vi "PowerMonitor Engine Driver.vi"(11 "Sequence Context":T2) -> (0 "error out":errorcluster)   [LabVIEW 2023, in "LTT_TeststandSteptypes.lvlib"]
uses:
  LTT_TeststandSteptypes.lvlib
  <vilib>/addons/TestStand/_TSLegacy.llb/LabVIEW Test - Sequence Context.ctl
  HardwareAbstractionLayer_LVOOP/Digital Input/DI_class/DI DAQ/Control/DI Step Control.ctl
  HardwareAbstractionLayer_LVOOP/PowerSupply/Control/PPS FGV Option.ctl
  Control/PowerData.ctl
  HardwareAbstractionLayer_LVOOP/Report/Report_class/Control/All Log Details.ctl
  HardwareAbstractionLayer_LVOOP/Report/Report_class/Control/UUT Test Info.ctl
  HardwareAbstractionLayer_LVOOP/Report/Report_class/Control/FE FRAME LOG.ctl
  HardwareAbstractionLayer_LVOOP/Report/Report_class/Control/FF FRAME LOG.ctl
  HardwareAbstractionLayer_LVOOP/Report/Report_class/Control/LIMIT TABLE.ctl
  HardwareAbstractionLayer_LVOOP/Report/Report_class/Control/ERROR LOG APPEND.ctl
  HardwareAbstractionLayer_LVOOP/Report/Report_class/Control/ERROR LOG.ctl
  HardwareAbstractionLayer_LVOOP/Report/Report_class/Control/FA FRAME LOG.ctl
  HardwareAbstractionLayer_LVOOP/Report/Report_class/Control/TEST RESULT LOG APPEND.ctl
  HardwareAbstractionLayer_LVOOP/Report/Report_class/Control/TEST RESULT LOG.ctl
  HardwareAbstractionLayer_LVOOP/Report/Report_class/Control/SYSTEM LOG.ctl
  HardwareAbstractionLayer_LVOOP/Report/Report_class/Control/Temperature LOG.ctl
  HardwareAbstractionLayer_LVOOP/Report/Report_class/Control/POWER STATUS.ctl
  HardwareAbstractionLayer_LVOOP/Report/Report_class/Control/CYCLE_DURATION_LOG.ctl
  Control/TimerStates.ctl
  GlobalVariable/GlobalVariableData.vi
  <vilib>/addons/TestStand/_TSUtility.llb/TestStand - Get Property Value (Number {Unsigned 32-bit Integer}).vi
  HardwareAbstractionLayer_LVOOP/Report/Report_class/Report.lvclass
  HardwareAbstractionLayer_LVOOP/Database/Database.lvclass
  HardwareAbstractionLayer_LVOOP/PowerSupply/PowerSupply.lvclass
  HardwareAbstractionLayer_LVOOP/Digital Input/DI_class/DI.lvclass
panel:
  in  "DI In":T1
  in  "stop":bool
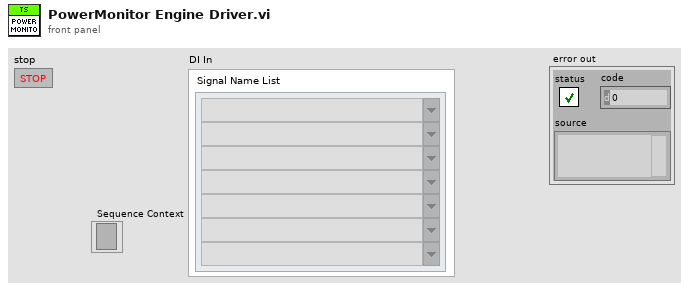
[diagram p1: front panel]
types:
  T1 = typedef "HardwareAbstractionLayer_LVOOP.lvlib/DI.lvclass/DI Step Control.ctl" = cluster{"Signal Name List":string[]}
  T2 = typedef "LabVIEW Test - Sequence Context.ctl" = refnum<k7>
  T3 = typedef "HardwareAbstractionLayer_LVOOP.lvlib/PowerSupply.lvclass/PPS FGV Option.ctl" = enum16{"Init Ref", "Get Ref", "Set Ref"}
  T4 = typedef "LTT_TeststandSteptypes.lvlib/PowerData.ctl" = cluster{"Chamber IP Ping":bool, "RAW_Power_Status":bool, "PDU1_Status_Instrument_Rack":bool, "PDU2_Status_PowerSupply_Rack_1":bool, "PDU3_Status_PowerSupply_Rack_2":bool}
  T5 = typedef "LTT_TeststandSteptypes.lvlib/TimerStates.ctl" = enum16{"Run", "Pause", "Reset"}
  T6 = typedef "HardwareAbstractionLayer_LVOOP.lvlib/Report.lvclass/All Log Details.ctl" = cluster{"UUT_TEST_INFO":T7, "FE_FRAME_LOG":T8, "FF_FRAME_LOG":T9, "LIMIT_TABLE":T10, "ERROR LOG Append":T11, "FA_FRAME_LOG":T13, "Socket No":u16, "TEST RESULT LOG Append":T14, "SYSTEM_LOG":T16, "Temperature log":T17, "POWER_STATUS":T18, "CYCLE_DURATION_LOG":T19}
  T7 = typedef "HardwareAbstractionLayer_LVOOP.lvlib/Report.lvclass/UUT Test Info.ctl" = cluster{"ID":string, "STATION_ID":string, "TEST_SOCKET_INDEX":string, "UUT_SERIAL_NUMBER":string, "TSW_VER":string, "VAL_SW_VER":string, "PROJECT_NAME":string, "PRODUCT_NAME":string, "PRODUCT_VARIANT":string, "TEST_NAME":string, "TEST_PHASE":string, "TEST_DESCRIPTION":string, "TEMP_CHAMBER_NAME":string, "START_DATE_TIME":string, "STOP_DATE_TIME ":string, "START_CYCLE_COUNT":string, "STOP_CYCLE_COUNT":string, "EXECUTION_TIME":string, "UUT_STATUS":string, "UUT_ERROR_CODE":string, "UUT_ERROR_MESSAGE":string, "TEST_SEQUENCE":string}
  T8 = typedef "HardwareAbstractionLayer_LVOOP.lvlib/Report.lvclass/FE FRAME LOG.ctl" = cluster{"ID":string, "UUT_TEST_INFO":string, "DATE_TIME":string, "CYCLE_NUMBER":string, "TEST_MODE":string, "CHAMBER_TEMP":string, "CAN_FRAME_RX":string, "Test Mode":u32, "LV_PPS_VOLTAGE":string, "LV_PPS_CURRENT":string, "HV_PPS_VOLTAGE":string, "HV_PPS_CURRENT":string, "SOCKET_NUMBER":string, "CAN_FRAME_RX_NO_OFF_BYTE":string}
  T9 = typedef "HardwareAbstractionLayer_LVOOP.lvlib/Report.lvclass/FF FRAME LOG.ctl" = cluster{"ID":string, "UUT_TEST_INFO":string, "DATE_TIME":string, "CYCLE_NUMBER":string, "TEST_MODE":string, "CAN_FRAME_RX":string, "CHAMBER_TEMP":string, "TestMode":u32, "SOCKET_NUMBER":string, "CAN_FRAME_RX_NO_OFF_BYTE":string}
  T10 = typedef "HardwareAbstractionLayer_LVOOP.lvlib/Report.lvclass/LIMIT TABLE.ctl" = cluster{"ID":string, "PRODUCT_NAME":string, "PRODUCT_VARIANT":string, "TEST_MODE":string, "PARAMETER_NAME":string, "COMPARISON_TYPE":string, "LOW_LIMIT":string, "HIGH_LIMIT":string, "UNIT":string, "ERROR_MESSSAGE":string, "SEVERITY":string}
  T11 = typedef "HardwareAbstractionLayer_LVOOP.lvlib/Report.lvclass/ERROR LOG APPEND.ctl" = T12[]
  T12 = typedef "HardwareAbstractionLayer_LVOOP.lvlib/Report.lvclass/ERROR LOG.ctl" = cluster{"ID":string, "UUT_TEST_INFO":string, "DATE_TIME":string, "CYCLE_NUMBER":string, "TEST_MODE":string, "SIGNAL_NAME":string, "SIGNAL_VALUE":string, "UNIT":string, "COMPARISON_VALUE":string, "ERROR_MESSAGE":string, "FRAME_TYPE":string, "LIMITID":string, "SOCKET_NUMBER":string}
  T13 = typedef "HardwareAbstractionLayer_LVOOP.lvlib/Report.lvclass/FA FRAME LOG.ctl" = cluster{"UUT_TEST_INFO":string, "CAN_FRAME_RX":string, "CAN_FRAME_RX_NO_OFF_BYTE":string}
  T14 = typedef "HardwareAbstractionLayer_LVOOP.lvlib/Report.lvclass/TEST RESULT LOG APPEND.ctl" = T15[]
  T15 = typedef "HardwareAbstractionLayer_LVOOP.lvlib/Report.lvclass/TEST RESULT LOG.ctl" = cluster{"ID":string, "UUT_TEST_INFO":string, "DATE_TIME":string, "CYCLE_NUMBER":string, "TEST_MODE":string, "SIGNAL_NAME":string, "SIGNAL_VALUE":string, "COMPARISON_VALUE":string, "ERROR_MESSAGE":string, "FRAME_TYPE":string, "LIMITID":string, "TEST_RESULT":string, "SOCKET_NUMBER":string}
  T16 = typedef "HardwareAbstractionLayer_LVOOP.lvlib/Report.lvclass/SYSTEM LOG.ctl" = cluster{"ID ":string, "DATE_TIME":string, "CYCLE_NUMBER":string, "TEST_MODE":string, "ERROR_MESSAGE":string}
  T17 = typedef "HardwareAbstractionLayer_LVOOP.lvlib/Report.lvclass/Temperature LOG.ctl" = cluster{"TEST_MODE":string, "CYCLE_NUMBER":string, "TEMPERATURE":cluster{"LV_PPS_TEMPERATURE":dbl, "HV_PPS1_TEMPERATURE":dbl, "HV_PPS2_TEMPERATURE":dbl, "HV_PPS3_TEMPERATURE":dbl, "HV_PPS4_TEMPERATURE":dbl, "HV_PPS5_TEMPERATURE":dbl, "HV_PPS6_TEMPERATURE":dbl, "CHAMBER_TEMPERATURE":dbl, "LOAD_U1_TEMPERATURE":dbl, "LOAD_V1_TEMPERATURE":dbl, "LOAD_W1_TEMPERATURE":dbl, "LOAD_U2_TEMPERATURE":dbl, "LOAD_V2_TEMPERATURE":dbl, "LOAD_W2_TEMPERATURE":dbl, "LOAD_U3_TEMPERATURE":dbl, "LOAD_V3_TEMPERATURE":dbl, "LOAD_W3_TEMPERATURE":dbl}, "Temperature Inrange":cluster{"LVPPS_Trip?":bool, "HVPPS1_Trip?":bool, "HVPPS2_Trip?":bool, "HVPPS3_Trip?":bool, "HVPPS4_Trip?":bool, "HVPPS5_Trip?":bool, "HVPPS6_Trip?":bool, "Chamber_Trip?":bool}}
  T18 = typedef "HardwareAbstractionLayer_LVOOP.lvlib/Report.lvclass/POWER STATUS.ctl" = cluster{"TEST_MODE":string, "CYCLE_NUMBER":string, "TYPE_POWER":string, "STATE":string}
  T19 = typedef "HardwareAbstractionLayer_LVOOP.lvlib/Report.lvclass/CYCLE_DURATION_LOG.ctl" = cluster{"CYCLE_NUMBER":string}
  T20 = typedef "HardwareAbstractionLayer_LVOOP.lvlib/Report.lvclass/Result FGV Data.ctl" = cluster{"Project Name":string, "Product Name":string, "Product Varient":string, "Test Name":string, "Test Phase":string, "Test Description":string, "Temp Chamber Name":string, "Schema":string, "Total No of Cycles":u32, "Current Cycle Number":u32, "Cycle Duration":u32, "Current Test Mode":string}
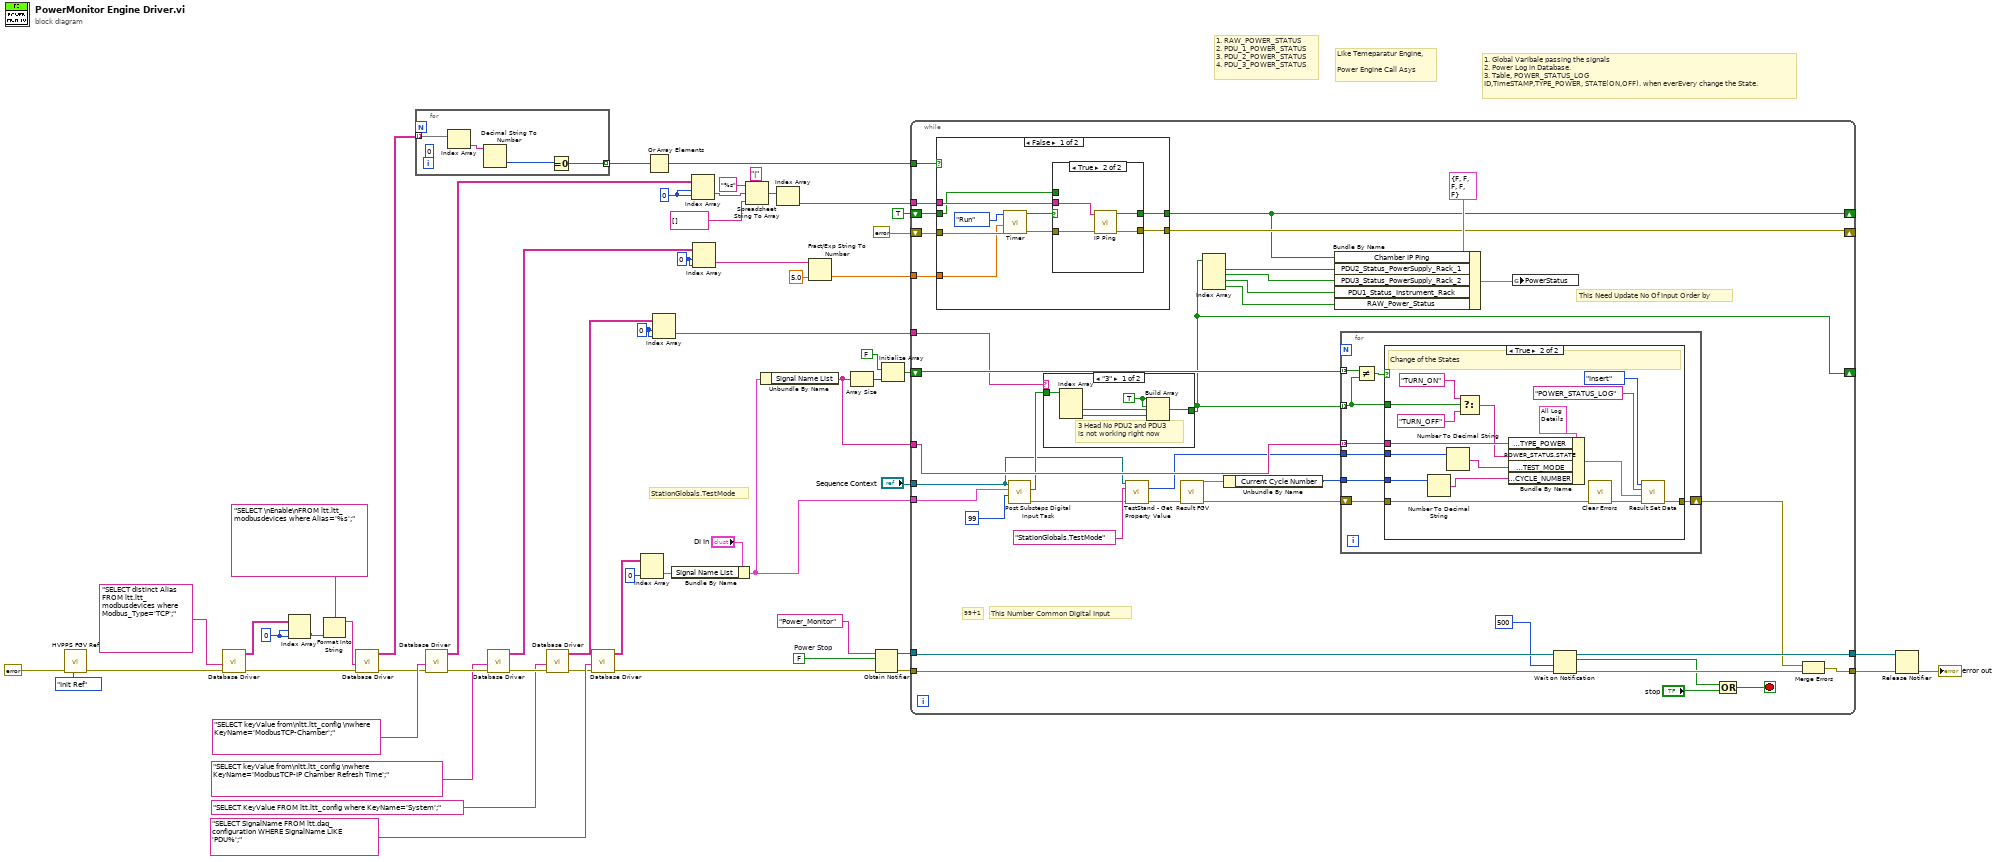
[diagram p0: block diagram]
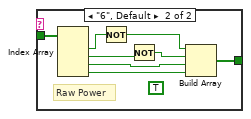
[diagram p2: hidden frame]
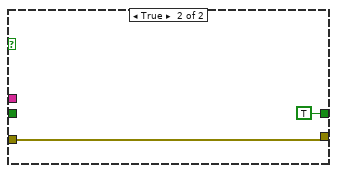
[diagram p4: hidden frame]
diagram:
  w6 = 0 ("index (row)")
  w19 = 0 ("disabled index (col)")
  w26 = 0 ("index (row)")
  w31 = 0 ("index (row)")
  w55 = FALSE  # Power Stop
  # "StationGlobals.TestMode"
  # "1. RAW_POWER_STATUS\n2. PDU_1_POWER_STATUS\n3. PDU_2_POWER_STATUS\n4. PDU_3_POWER_STATUS"
  # "Like Temeparatur Engine,\n\nPower Engine Call Asys"
  # "1. Global Varibale passing the signals\n2. Power Log in Database.\n3. Table, POWER_STATUS_LOG\nID,TimeSTAMP,TYPE_POWER, STATE(ON,OFF). when everEvery change the State."
  n1 = call "HVPPS FGV Ref.vi"("Option"=PPS_FGV_Option."Init Ref", "error in"=errorcluster {"status"=FALSE, "code"=0, "source"=""} ("error in (no error)")) -> ("error out"=w2:errorcluster)  [unwired: 8 in, 1 out]
  n2 = call "Database Driver.vi"("error in"=w2, "SQL query"="SELECT distinct Alias FROM ltt.ltt_modbusdevices where Modbus_Type='TCP';") -> ("error out"=w13:errorcluster, "data"=w20:string[][])  [unwired: 6 in, 2 out]
  n3 = Index Array(array=w20, index (row)=w19, index (col)=w19) -> (element=w14:string)
  n4 = Format Into String(format string="SELECT \nEnable\nFROM ltt.ltt_modbusdevices where Alias='%s';", w14) -> (resulting string=w17:string)  [unwired: 2 in, 1 out]
  n5 = call "Database Driver.vi"("error in"=w13, "SQL query"=w17) -> ("error out"=w12:errorcluster, "data"=w16:string[][])  [unwired: 6 in, 2 out]
  n6 = for {
    tunnel: w16 -> [w61] mode=indexing
    tunnel: [w58] -> w11 mode=indexing
    (unwired) 0 ("disabled index (col)")
    n7 = Index Array(array=w61) -> (element=w60:string)  [unwired: 1 in]
    n8 = Decimal String To Number(string=w60) -> (number=w59:i32)  [unwired: 2 in, 1 out]
    n9 = Equal To 0?(x=w59) -> (x = 0?=w58:bool)
  }
  n10 = call "Database Driver.vi"("error in"=w12, "SQL query"="SELECT keyValue from\nltt.ltt_config \nwhere KeyName='ModbusTCP-Chamber';") -> ("error out"=w29:errorcluster, "data"=w32:string[][])  [unwired: 6 in, 2 out]
  n11 = call "Database Driver.vi"("error in"=w29, "SQL query"="SELECT keyValue from\nltt.ltt_config \nwhere KeyName='ModbusTCP-IP Chamber Refresh Time';") -> ("error out"=w10:errorcluster, "data"=w27:string[][])  [unwired: 6 in, 2 out]
  n12 = call "Database Driver.vi"("error in"=w10, "SQL query"="SELECT KeyValue FROM ltt.ltt_config where KeyName='System';") -> ("error out"=w9:errorcluster, "data"=w7:string[][])  [unwired: 6 in, 2 out]
  n13 = call "Database Driver.vi"("error in"=w9, "SQL query"="SELECT SignalName FROM ltt.daq_configuration WHERE SignalName LIKE 'PDU%';") -> ("error out"=w43:errorcluster, "data"=w45:string[][])  [unwired: 6 in, 2 out]
  n14 = Index Array(array=w45, index (col)=0 ("disabled index (col)")) -> (element=w41:string[])  [unwired: 1 in]
  n15 = Or Array Elements(Boolean array=w11) -> (logical OR=w4:bool)
  n16 = Index Array(array=w7, index (row)=w6, index (col)=w6) -> (element=w5:string)
  n17 = Bundle By Name(cluster="DI In", "Signal Name List"=w41) -> (w40:T1)
  n18 = Index Array(array=w32, index (row)=w31, index (col)=w31) -> (element=w38:string)
  n19 = Index Array(array=w27, index (row)=w26, index (col)=w26) -> (element=w25:string)
  n20 = Spreadsheet String To Array(delimiter (Tab)="|" ("format string"), format string="%s", spreadsheet string=w38, array type (2D Dbl)=string[] []) -> (array=w36:string[])
  n21 = Unbundle By Name(w40) -> ("Signal Name List"=w49:string[])
  n22 = Index Array(array=w36) -> (element=w30:string)  [unwired: 1 in]
  n23 = Fract/Exp String To Number(string=w25, default (0 dbl)=5.0 ("default (0 DBL)")) -> (number=w23:dbl)  [unwired: 2 in, 1 out]
  n24 = Array Size(array=w49) -> (size(s)=w48:i32)
  n25 = Obtain Notifier(name (unnamed)="Power_Monitor", notification data type=w55, error in (no error)=w43) -> (notifier out=w53:refnum<notifier>, error out=w54:errorcluster)  [unwired: 1 in, 1 out]
  n26 = Initialize Array(FALSE, w48) -> (w46:bool[])
  n27 = while {
    tunnel: w54 -> [w93]
    tunnel: [w86] -> w52
    tunnel: "Sequence Context" -> [w75]
    tunnel: w53 -> [w91]
    tunnel: [w89] -> w50
    tunnel: w40 -> [w83]
    shift-right: [w78] -> _
    shift-left: w46 -> [w81]
    tunnel: w49 -> [w82]
    tunnel: w30 -> [w68]
    tunnel: w23 -> [w67]
    shift-right: [w64] -> _
    shift-left: TRUE ("Sucessful?") -> [w66]
    shift-right: [w65] -> _
    shift-left: errorcluster {"status"=FALSE, "code"=0, "source"=""} ("error in") -> [w69]
    tunnel: w4 -> [w63]
    tunnel: w5 -> [w62]
    stop <- w88 stop-if-true
    # "99+1"
    # "This Need Update No Of Input Order by"
    # "This Number Common Digital Input"
    n28 = case shown="False" w63 {
      tunnel: w69 -> [w119 w129]
      tunnel: w68 -> [w117 _]
      tunnel: w67 -> [w116 _]
      tunnel: w66 -> [w115 _]
      tunnel: [w114 w129] -> w65
      tunnel: [w113 TRUE ("Sucessful?")] -> w64
      frame False {
        n29 = call "Timer.vi"("error in"=w119, "Refresh Time"=w116, "Options"=TimerStates."Run") -> ("error out"=w121:errorcluster, "Refresh"=w120:bool)  [unwired: 6 in, 1 out]
        n30 = case shown="True" w120 {
          tunnel: w121 -> [w123 w127]
          tunnel: w117 -> [_ w126]
          tunnel: [w122 w125] -> w113
          tunnel: [w123 w124] -> w114
          tunnel: w115 -> [w122 _]
          frame False {
          }
          frame True {
            n31 = call "IP Ping.vi"("error in (no error)"=w127, "IP/Address"=w126) -> ("error out"=w124:errorcluster, "Sucessful?"=w125:bool)  [unwired: 8 in]
          }
        }
      }
      frame True {
      }
    }
    n32 = call "Post Substeps Digital Input Task.vi"("Socket No"=u16 99, "DI In"=w83, "Sequence Context In"=w75) -> ("error out"=w76:errorcluster, "DigitalInputRead"=w79:bool[])  [unwired: 5 in, 2 out]
    n33 = case shown="\"3\"" w62 {
      tunnel: w79 -> [w104 w112]
      tunnel: [w101 w111] -> w78
      frame "3" {
        w100 = TRUE ("element")
        # "3 Head No PDU2 and PDU3\nis not working right now"
        n34 = Index Array(array=w104) -> (element #2=w103:bool, element #3=w102:bool)  [unwired: 3 in, 1 out]
        n35 = Build Array(w100, w100, w103, w102) -> (w101:bool[])
      }
      frame "6", Default {
        (unwired) TRUE
        # "Raw Power"
        n36 = Index Array(array=w112) -> (element #1=w110:bool, element #2=w109:bool, element #3=w106:bool, element #4=w105:bool)  [unwired: 4 in]
        n37 = Not(x=w110) -> (.not. x?=w107:bool)
        n38 = Not(x=w109) -> (.not. x?=w108:bool)
        n39 = Build Array(w107, w108, w106, w105) -> (w111:bool[])
      }
    }
    n40 = call-poly <vilib>:"TestStand - Get Property Value.vi"("Sequence Context In"=w75, "Lookup String"="StationGlobals.TestMode", "error in (no error)"=w76) -> ("Value"=w74:u32, "error out"=w73:errorcluster)  [unwired: 10 in, 1 out]
    n41 = call "Result FGV.vi"("error in"=w73) -> ("error out"=w72:errorcluster, "Result FGV Data Out"=w71:T20)  [unwired: 9 in]
    n42 = Index Array(array=w78) -> (element #1=w97:bool, element #2=w96:bool, element #3=w95:bool, element #4=w94:bool)  [unwired: 4 in]
    n43 = Unbundle By Name(w71) -> ("Current Cycle Number"=w70:u32)
    n44 = Bundle By Name(cluster=T4 {"Chamber IP Ping"=FALSE, "RAW_Power_Status"=FALSE, "PDU1_Status_Instrument_Rack"=FALSE, "PDU2_Status_PowerSupply_Rack_1"=FALSE, "PDU3_Status_PowerSupply_Rack_2"=FALSE} ("PowerData"), "Chamber IP Ping"=w64, "PDU2_Status_PowerSupply_Rack_1"=w97, "PDU3_Status_PowerSupply_Rack_2"=w96, "PDU1_Status_Instrument_Rack"=w95, "RAW_Power_Status"=w94) -> (w98:T4)
    n45 = for {
      shift-right: [w136] -> w85
      shift-left: w72 -> [w137]
      tunnel: w78 -> [w132] mode=indexing
      tunnel: w82 -> [w135] mode=indexing
      tunnel: w81 -> [w134] mode=indexing
      tunnel: w74 -> [w131]
      tunnel: w70 -> [w130]
      n46 = Not Equal?(x=w134, y=w132) -> (x != y?=w133:bool)
      n47 = case shown="True" w133 {
        tunnel: w137 -> [w138 w154]
        tunnel: [w138 w153] -> w136
        tunnel: w135 -> [_ w148]
        tunnel: w132 -> [_ w145]
        tunnel: w131 -> [_ w143]
        tunnel: w130 -> [_ w140]
        frame False {
        }
        frame True {
          # "Change of the States"
          n48 = Number To Decimal String(number=w140) -> (decimal integer string=w139:string)  [unwired: 1 in]
          n49 = Number To Decimal String(number=w143) -> (decimal integer string=w142:string)  [unwired: 1 in]
          n50 = Select(t="TURN_ON" ("POWER_STATUS.STATE"), s=w145, f="TURN_OFF" ("POWER_STATUS.STATE")) -> (s? t:f=w144:string)
          n51 = Bundle By Name(cluster=T6 {"UUT_TEST_INFO"={"ID"="", "STATION_ID"="", "TEST_SOCKET_INDEX"="", "UUT_SERIAL_NUMBER"="", "TSW_VER"="", "VAL_SW_VER"="", "PROJECT_NAME"="", "PRODUCT_NAME"="", "PRODUCT_VARIANT"="", "TEST_NAME"="", "TEST_PHASE"="", "TEST_DESCRIPTION"="", "TEMP_CHAMBER_NAME"="", "START_DATE_TIME"="", "STOP_DATE_TIME "="", "START_CYCLE_COUNT"="", "STOP_CYCLE_COUNT"="", "EXECUTION_TIME"="", "UUT_STATUS"="", "UUT_ERROR_CODE"="", "UUT_ERROR_MESSAGE"="", "TEST_SEQUENCE"=""}, "FE_FRAME_LOG"={"ID"="", "UUT_TEST_INFO"="", "DATE_TIME"="", "CYCLE_NUMBER"="", "TEST_MODE"="", "CHAMBER_TEMP"="", "CAN_FRAME_RX"="", "Test Mode"=0, "LV_PPS_VOLTAGE"="", "LV_PPS_CURRENT"="", "HV_PPS_VOLTAGE"="", "HV_PPS_CURRENT"="", "SOCKET_NUMBER"="", "CAN_FRAME_RX_NO_OFF_BYTE"=""}, "FF_FRAME_LOG"={"ID"="", "UUT_TEST_INFO"="", "DATE_TIME"="", "CYCLE_NUMBER"="", "TEST_MODE"="", "CAN_FRAME_RX"="", "CHAMBER_TEMP"="", "TestMode"=0, "SOCKET_NUMBER"="", "CAN_FRAME_RX_NO_OFF_BYTE"=""}, "LIMIT_TABLE"={"ID"="", "PRODUCT_NAME"="", "PRODUCT_VARIANT"="", "TEST_MODE"="", "PARAMETER_NAME"="", "COMPARISON_TYPE"="", "LOW_LIMIT"="", "HIGH_LIMIT"="", "UNIT"="", "ERROR_MESSSAGE"="", "SEVERITY"=""}, "ERROR LOG Append"=[], "FA_FRAME_LOG"={"UUT_TEST_INFO"="", "CAN_FRAME_RX"="", "CAN_FRAME_RX_NO_OFF_BYTE"=""}, "Socket No"=1, "TEST RESULT LOG Append"=[], "SYSTEM_LOG"={"ID "="", "DATE_TIME"="", "CYCLE_NUMBER"="", "TEST_MODE"="", "ERROR_MESSAGE"=""}, "Temperature log"={"TEST_MODE"="", "CYCLE_NUMBER"="", "TEMPERATURE"={"LV_PPS_TEMPERATURE"=0.0, "HV_PPS1_TEMPERATURE"=0.0, "HV_PPS2_TEMPERATURE"=0.0, "HV_PPS3_TEMPERATURE"=0.0, "HV_PPS4_TEMPERATURE"=0.0, "HV_PPS5_TEMPERATURE"=0.0, "HV_PPS6_TEMPERATURE"=0.0, "CHAMBER_TEMPERATURE"=0.0, "LOAD_U1_TEMPERATURE"=0.0, "LOAD_V1_TEMPERATURE"=0.0, "LOAD_W1_TEMPERATURE"=0.0, "LOAD_U2_TEMPERATURE"=0.0, "LOAD_V2_TEMPERATURE"=0.0, "LOAD_W2_TEMPERATURE"=0.0, "LOAD_U3_TEMPERATURE"=0.0, "LOAD_V3_TEMPERATURE"=0.0, "LOAD_W3_TEMPERATURE"=0.0}, "Temperature Inrange"={"LVPPS_Trip?"=FALSE, "HVPPS1_Trip?"=FALSE, "HVPPS2_Trip?"=FALSE, "HVPPS3_Trip?"=FALSE, "HVPPS4_Trip?"=FALSE, "HVPPS5_Trip?"=FALSE, "HVPPS6_Trip?"=FALSE, "Chamber_Trip?"=FALSE}}, "POWER_STATUS"={"TEST_MODE"="", "CYCLE_NUMBER"="", "TYPE_POWER"="", "STATE"=""}, "CYCLE_DURATION_LOG"={"CYCLE_NUMBER"=""}} ("Set Data"), "POWER_STATUS.TYPE_POWER"=w148, "POWER_STATUS.STATE"=w144, "POWER_STATUS.TEST_MODE"=w142, "POWER_STATUS.CYCLE_NUMBER"=w139) -> (w152:T6)
          n52 = call <vilib>:"Clear Errors.vi"("error in (no error)"=w154) -> ("error out"=w141:errorcluster)  [unwired: 5 in, 1 out]
          n53 = call "Result Set Data.vi"("error in"=w141, "Set Data"=w152, "Table Name"="POWER_STATUS_LOG", "Action"=enum16{"Insert", "Update"}."Insert") -> ("error out"=w153:errorcluster)  [unwired: 7 in]
        }
      }
    }
    n54 = global write "GlobalVariableData.vi" "PowerStatus"(w98) -> ()
    n55 = Wait on Notification(notifier=w91, timeout in ms (-1)=500, error in (no error)=w93) -> (notifier out=w89:refnum<notifier>, notification=w90:bool, error out=w92:errorcluster)  [unwired: 1 in, 1 out]
    n56 = Compound Arithmetic op=OR(w90, "stop") -> (w88:bool)
    n57 = Merge Errors(w85, w92) -> (w86:errorcluster)
  }
  n58 = Release Notifier(notifier=w50, error in (no error)=w52) -> (error out=→"error out":errorcluster)  [unwired: 1 in, 2 out]
